vi "Close.vi"(8 "error in (no error)":errorcluster, 10 "write if changed (T)":bool=TRUE, 11 "Ini-File in":refnum<class "Ini-File.lvclass">) -> (0 "error out":errorcluster, 3 "Ini-File out":refnum<class "Ini-File.lvclass">)   [LabVIEW 2013, in "Configuration.lvlib" / "Ini-File.lvclass"]
doc: "Close connection to ini-file."
uses:
  Ini-File.lvclass
  <vilib>/Utility/config.llb/Config Data RefNum.ctl
  Ini-File.lvclass/Ini-File.ctl
  <vilib>/Utility/config.llb/NI_LVConfig.lvlib
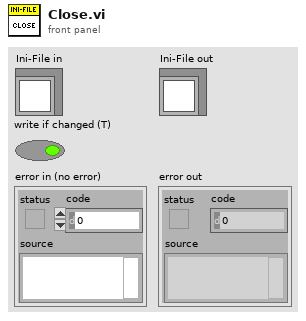
[diagram p1: front panel]
types:
  T1 = typedef "NI_LVConfig.lvlib/Config Data RefNum.ctl" = refnum<k1>
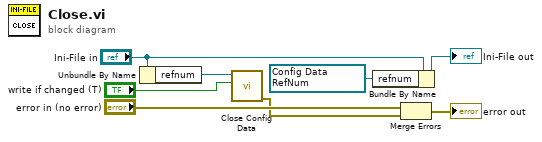
[diagram p0: block diagram]
diagram:
  w3 = T1 refnum items=["config data"] ("refnum")
  n1 = Unbundle By Name("Ini-File in") -> ("refnum"=w7:T1)
  n2 = call <vilib>:"Close Config Data.vi"("write file if changed (T)"="write if changed (T)", "refnum"=w7) -> ("error out"=w5:errorcluster)  [unwired: 8 in, 1 out]
  n3 = Bundle By Name(cluster="Ini-File in", "refnum"=w3) -> (→"Ini-File out":refnum<class "Ini-File.lvclass">)
  n4 = Merge Errors("error in (no error)", w5) -> (→"error out":errorcluster)
